vi "Decimator.vi"(8 "Decimator":i32, 11 "Array In":dbl[][](array[numeric])) -> (3 "DecimatedArrayOut":dbl[][](array[numeric]))   [LabVIEW 2022 SP3]
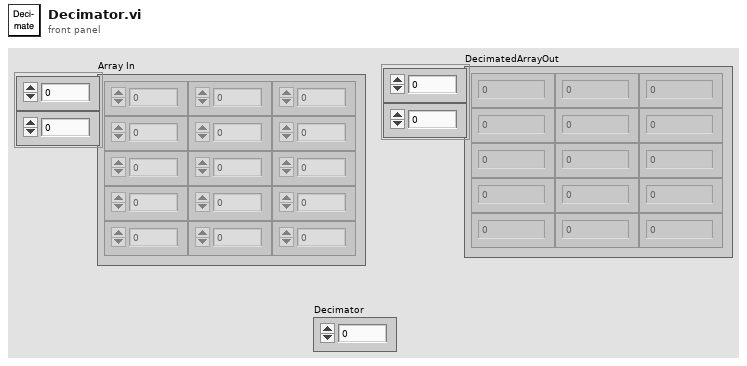
[diagram p1: front panel]
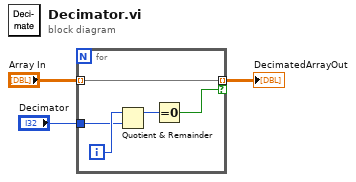
[diagram p0: block diagram]
diagram:
  n1 = for {
    tunnel: "Array In" -> [w5] mode=indexing
    tunnel: "Decimator" -> [w7]
    tunnel: [w5] -> w2 mode=indexing if=w4
    i -> [w8]
    n2 = Quotient & Remainder(x=w8, y=w7) -> (x-y*floor(x/y)=w6:i32)  [unwired: 1 out]
    n3 = Equal To 0?(x=w6) -> (x = 0?=w4:bool)
  }
  "DecimatedArrayOut" <- w2
